vi "loop_data_labels.vi"() -> (0 "Loop Data Labels":string[](array[string])=["Timestamp", "Vap Mass Flow", "Liq Mass Flow", "DP", "Liq Tank P", "LiqTank T", "Sep P", "SepT", "Liq In P", "Liq In T", "Vap Tank P", "Vap Tank T", "Dev Section P", "Dev Section T", "Up TS P", "Up TS T", "Low TS P", "Low TS T", "Cond Top T", "Evap Top T", "Cond Bot T", "Evap Bot T", "Win 3-4 P", "Top Heat T", "Bot Heat T", ""])   [LabVIEW 2017]
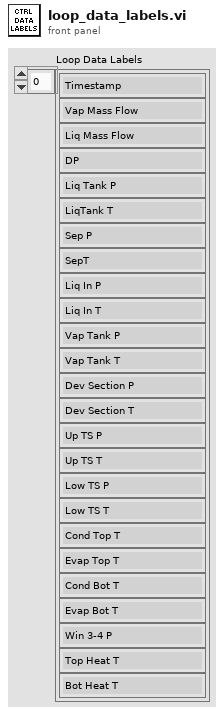
[diagram p1: front panel]
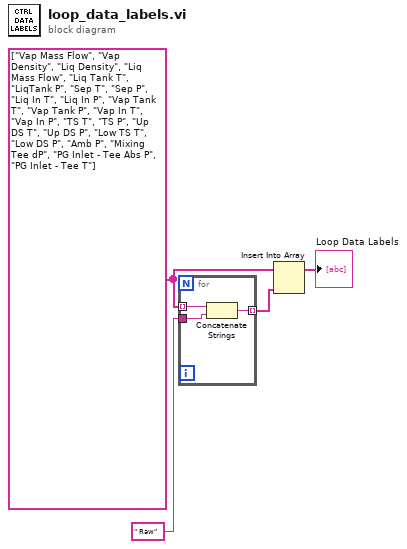
[diagram p0: block diagram]
diagram:
  w1 = string[] ["Vap Mass Flow", "Vap Density", "Liq Density", "Liq Mass Flow", "Liq Tank T", "LiqTank P", "Sep T", "Sep P", "Liq In T", "Liq In P", "Vap Tank T", "Vap Tank P", "Vap In T", "Vap In P", "TS T", "TS P", "Up DS T", "Up DS P", "Low TS T", "Low DS P", "Amb P", "Mixing Tee dP", "PG Inlet - Tee Abs P", "PG Inlet - Tee T"] ("subarray")
  n1 = for {
    tunnel: w1 -> [w7] mode=indexing
    tunnel: [w6] -> w4 mode=indexing
    tunnel: " Raw" ("string") -> [w5]
    n2 = Concatenate Strings(w7, w5) -> (w6:string)
  }
  n3 = Insert Into Array(array=w1, new element=w4) -> (→"Loop Data Labels":string[])  [unwired: 1 in]
